vi "Global_Init.vi"(11 "Object":T1) -> ()   [LabVIEW 2020, in "Project Provider.lvlib"]
uses:
  Project Provider.lvlib
  <resource>/Framework/Providers/API/ItemRef.ctl
  <resource>/Framework/Providers/API/mxLvOverlayAlias.ctl
panel:
  out "error out":errorcluster
  in  "error in":errorcluster
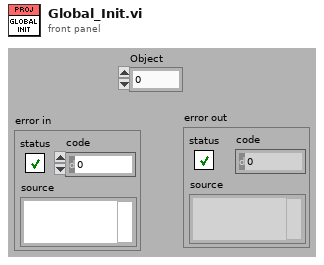
[diagram p1: front panel]
types:
  T1 = typedef "ItemRef.ctl" = u64
  T2 = typedef "mxLvOverlayAlias.ctl" = cluster{"Overlay Alias":string, "Icon File Name":path}
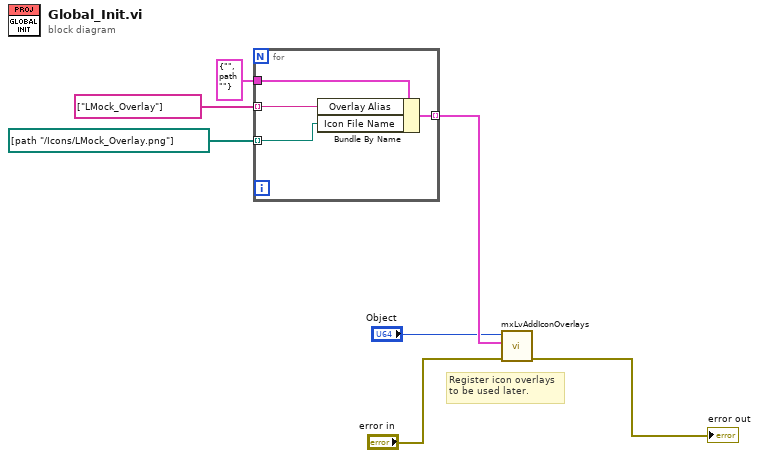
[diagram p0: block diagram]
diagram:
  # "Register icon overlays\nto be used later."
  n1 = for {
    tunnel: T2 {"Overlay Alias"="", "Icon File Name"=path ""} ("Icon Overlay Alias") -> [w11]
    tunnel: [w10] -> w6 mode=indexing
    tunnel: string[] ["LMock_Overlay"] ("overlay alias") -> [w9] mode=indexing
    tunnel: path[] [path "../Icons/LMock_Overlay.png"] ("icon filename") -> [w8] mode=indexing
    n2 = Bundle By Name(cluster=w11, "Overlay Alias"=w9, "Icon File Name"=w8) -> (w10:T2)
  }
  n3 = call <resource>:"mxLvAddIconOverlays.vi"("error in"="error in", "Overlay Aliases"=w6, "Item"="Object") -> ("error out"=→"error out":errorcluster)  [unwired: 7 in, 1 out]
